vi "Set Field value.vi"(0 "Field":dbl) -> ()   [LabVIEW 2021]
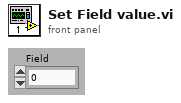
[diagram p1: front panel]
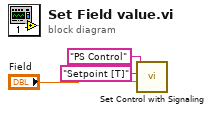
[diagram p0: block diagram]
diagram:
  n1 = call "Set Control with Signaling.vi"("Value"="Field", "Control Name"="Setpoint [T]", "VI Name"="PS Control") -> ()  [unwired: 8 in, 1 out]
